vi "ReadWrite.vi"(6 "Values":dbl[](array[numeric]), 7 "tdms file in":refnum<k34>, 8 "error in (no error)":errorcluster, 9 "Channel Refs":T1[](array[typedef]) format="%.0x", 10 "Wfm Refs":refnum<class "Single Waveform Read (DBL).lvclass">[](array[class]), 11 "Compiled.Settings":T2={"Name"="", "Async Init Timeout"=0, "File Data"={"Date Captured"="", "Directory"="", "Name"="", "Groups"=[], "Meta Data"=[]}, "Segment Files"=FALSE, "Segment Every"=0.0, "Trigger?"=FALSE, "Segment by"=enum."Size (MB)", "Trigger Ref"=0} {"Trigger Ref" format="%.0x"; "File Data"."Groups"."Channels"."Data Reference in" format="%.0x"}) -> (0 "error out":errorcluster, 1 "Bytes Written":u64, 2 "tdms file out":refnum<k34>, 3 "Compiled.Settings Out":T2={"Name"="", "Async Init Timeout"=0, "File Data"={"Date Captured"="", "Directory"="", "Name"="", "Groups"=[], "Meta Data"=[]}, "Segment Files"=FALSE, "Segment Every"=0.0, "Trigger?"=FALSE, "Segment by"=enum."Size (MB)", "Trigger Ref"=0} {"Trigger Ref" format="%.0x"; "File Data"."Groups"."Channels"."Data Reference in" format="%.0x"})   [LabVIEW 2023, in "Embedded TDMS Logger Engine.lvlib"]
uses:
  Embedded TDMS Logger Engine.lvlib
  Shared/Compiled.Settings.ctl
  Shared/FileData.ctl
  Shared/GroupData.ctl
  Shared/Meta Data Item.ctl
  Shared/ChannelData.ctl
  <vilib>/NI VeriStand/Custom Device API/Data Reference.ctl
  Shared/SegmentOptions.ctl
  <vilib>/NI VeriStand/Custom Device Waveform API/Single Waveform Read (DBL)/Single Waveform Read (DBL).lvclass
  C:/Program Files/National Instruments/LabVIEW 2023/vi.lib/NI VeriStand/Custom Device Waveform API/Waveform Session.lvclass
  <vilib>/NI VeriStand/Custom Device Waveform API/Waveform Session.lvclass/Waveform Session.ctl
  <vilib>/NI VeriStand/Custom Device Waveform API/Single Waveform Read (DBL)/Single Waveform Read (DBL).lvclass/Single Waveform Read (DBL).ctl
  <vilib>/NI VeriStand/Custom Device Waveform API/Internal Comm Classes/WPL Comm/WPL Comm (1D DBL)/WPL Comm (1D DBL).lvclass/WPL Comm (1D DBL).ctl
  <vilib>/NI VeriStand/Custom Device Waveform API/Single Waveform Read (DBL)/NI VeriStand - Read Single Waveform (DBL).vi
  <vilib>/NI VeriStand/Custom Device Waveform API/Internal Comm Classes/WPL Comm/WPL Comm (1D DBL)/Comm_read 1d dbl.vi
  <vilib>/NI VeriStand/Custom Device Waveform API/Check Opened.vi
  <vilib>/NI VeriStand/Custom Device Waveform API/Internal Comm Classes/WPL Comm/Convert Q Error to Shutdown Error.vi
  <vilib>/Utility/error.llb/Error Cluster From Error Code.vi
  <vilib>/NI VeriStand/Custom Device Waveform API/NI_VS Custom Device Waveform API.lvlib
  Shared/Embedded TDMS Logger Shared.lvlib
  <vilib>/NI VeriStand/Custom Device API/Custom Device API.lvlib
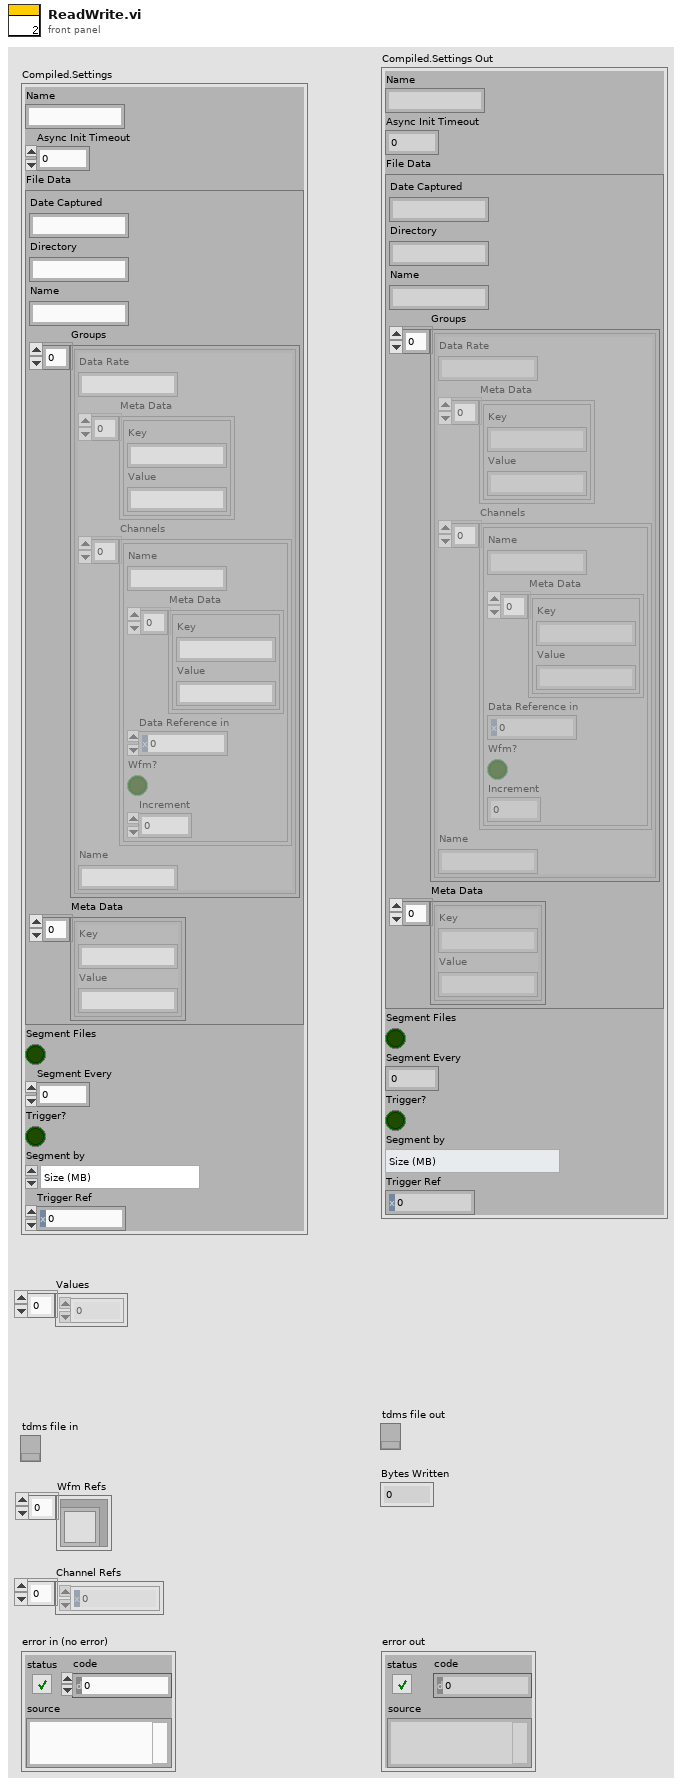
[diagram p1: front panel]
types:
  T1 = typedef "Custom Device API.lvlib/Data Reference.ctl" = i32
  T2 = typedef "Embedded TDMS Logger Shared.lvlib/Compiled.Settings.ctl" = cluster{"Name":string, "Async Init Timeout":u16, "File Data":T3, "Segment Files":bool, "Segment Every":dbl, "Trigger?":bool, "Segment by":T7, "Trigger Ref":T1}
  T3 = typedef "Embedded TDMS Logger Shared.lvlib/FileData.ctl" = cluster{"Date Captured":string, "Directory":string, "Name":string, "Groups":T4[], "Meta Data":T5[]}
  T4 = typedef "Embedded TDMS Logger Shared.lvlib/GroupData.ctl" = cluster{"Data Rate":string, "Meta Data":T5[], "Channels":T6[], "Name":string}
  T5 = typedef "Embedded TDMS Logger Shared.lvlib/Meta Data Item.ctl" = cluster{"Key":string, "Value":string}
  T6 = typedef "Embedded TDMS Logger Shared.lvlib/ChannelData.ctl" = cluster{"Name":string, "Meta Data":T5[], "Data Reference":T1, "Wfm?":bool, "Increment":dbl}
  T7 = typedef "SegmentOptions.ctl" = enum16{"Time (s)", "Size (MB)"}
  T8 = typedef "NI_VS Custom Device Waveform API.lvlib/Waveform properties.ctl" = cluster{"Data reference":T9, "t0 at start":timestamp, "dt":dbl, "offset from start (samples)":u64}
  T9 = typedef "Custom Device API.lvlib/Waveform Data Reference.ctl" = i32
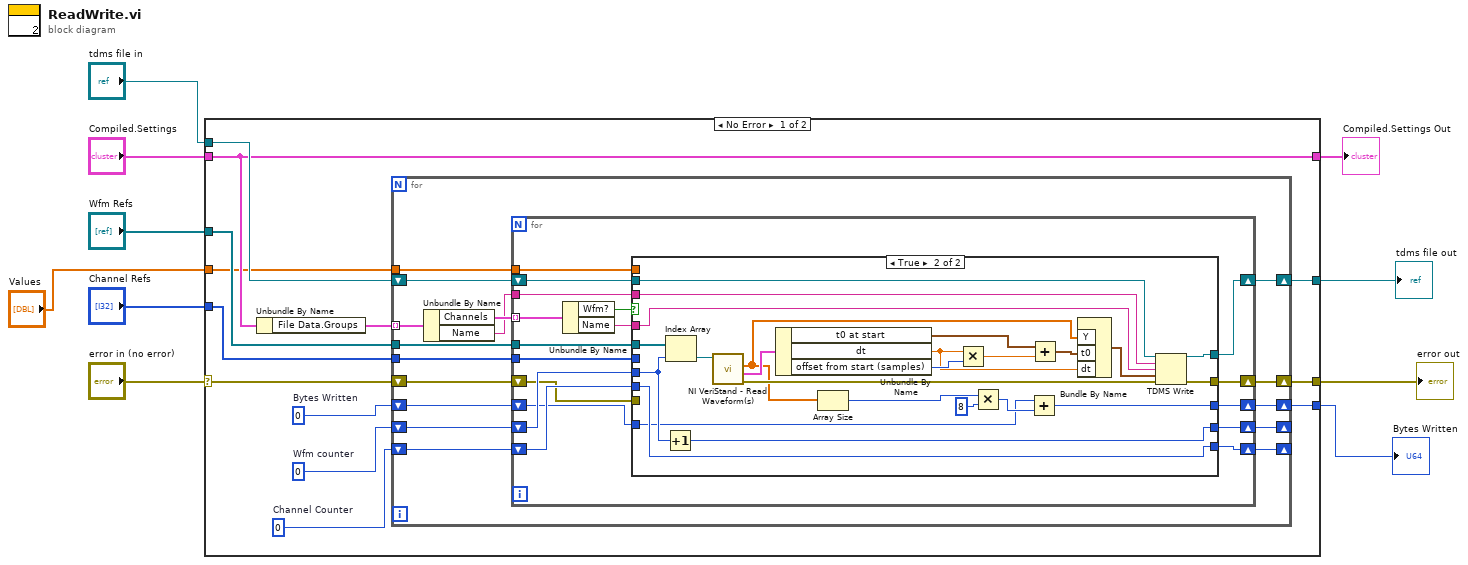
[diagram p0: block diagram]
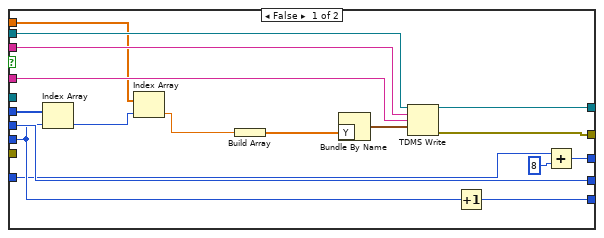
[diagram p2: hidden frame]
diagram:
  n1 = case shown="No Error" "error in (no error)" {
    selector: "error in (no error)" -> [w16 w99]
    tunnel: "Compiled.Settings" -> [w14 w98]
    tunnel: "tdms file in" -> [w22 w100]
    tunnel: [w21 w100] -> w7
    tunnel: "Wfm Refs" -> [w20 _]
    tunnel: "Channel Refs" -> [w17 _]
    tunnel: [w15 w99] -> w4
    tunnel: [w14 w98] -> w3
    tunnel: [w12 _] -> w2
    tunnel: "Values" -> [w11 _]
    frame No Error {
      w13 = u64 0  # Bytes Written
      w19 = 0  # Wfm counter
      w18 = 0  # Channel Counter
      n2 = Unbundle By Name(w14) -> ("File Data.Groups"=w23:T4[])
      n3 = for {
        tunnel: w23 -> [w39] mode=indexing
        shift-right: [w29] -> w21
        shift-left: w22 -> [w36]
        tunnel: w20 -> [w35]
        shift-right: [w32] -> _
        shift-left: w19 -> [w34]
        shift-right: [w31] -> _
        shift-left: w18 -> [w33]
        tunnel: w17 -> [w30]
        shift-right: [w28] -> w15
        shift-left: w16 -> [w27]
        shift-right: [w25] -> w12
        shift-left: w13 -> [w26]
        tunnel: w11 -> [w24]
        n4 = Unbundle By Name(w39) -> ("Channels"=w38:T6[], "Name"=w37:string)
        n5 = for {
          tunnel: w38 -> [w56] mode=indexing
          tunnel: w37 -> [w47]
          shift-right: [w45] -> w29
          shift-left: w36 -> [w54]
          tunnel: w35 -> [w53]
          shift-right: [w50] -> w32
          shift-left: w34 -> [w52]
          shift-right: [w49] -> w31
          shift-left: w33 -> [w51]
          tunnel: w30 -> [w48]
          shift-right: [w44] -> w28
          shift-left: w27 -> [w43]
          shift-right: [w41] -> w25
          shift-left: w26 -> [w42]
          tunnel: w24 -> [w40]
          n6 = Unbundle By Name(w56) -> ("Wfm?"=w55:bool, "Name"=w46:string)
          n7 = case shown="True" w55 {
            tunnel: w54 -> [w70 w97]
            tunnel: w53 -> [_ w95]
            tunnel: w52 -> [w73 w94]
            tunnel: w51 -> [w64 w92]
            tunnel: [w73 w93] -> w50
            tunnel: [w72 w92] -> w49
            tunnel: w48 -> [w71 _]
            tunnel: w47 -> [w69 w82]
            tunnel: w46 -> [w65 w81]
            tunnel: [w68 w90] -> w45
            tunnel: [w67 w91] -> w44
            tunnel: w43 -> [_ _]
            tunnel: w42 -> [w62 w78]
            tunnel: [w61 w77] -> w41
            tunnel: w40 -> [w58 _]
            frame False {
              n8 = Index Array(array=w71, index=w64) -> (element=w60:T1)
              n9 = Index Array(array=w58, index=w60) -> (element=w59:dbl)
              n10 = Build Array(w59) -> (w57:dbl[])
              n11 = Bundle By Name("Y"=w57) -> (w66:waveform(dbl))  [unwired: 1 in]
              n12 = TDMS Write(0:w70, 5:w69, 7:w65, 9:w66) -> (4:w68:refnum<k34>, 15:w67:errorcluster)  [unwired: 2 in, 2 out]
              n13 = Increment(x=w64) -> (x+1=w72:i32)
              n14 = Add(x=w62, y=u64 8) -> (x+y=w61:u64)
            }
            frame True {
              n15 = Increment(x=w94) -> (x+1=w93:i32)
              n16 = Index Array(array=w95, index=w94) -> (element=w96:refnum<class "Single Waveform Read (DBL).lvclass">)
              n17 = call-poly <vilib>:"NI VeriStand - Read Waveform(s).vi"("Single Waveform Read Session (DBL) in"=w96) -> ("error out"=w89:errorcluster, "Properties"=w88:T8, "Data"=w75:dbl[])  [unwired: 6 in, 2 out]
              n18 = Unbundle By Name(w88) -> ("t0 at start"=w76:timestamp, "dt"=w85:dbl, "offset from start (samples)"=w87:u64)
              n19 = Array Size(array=w75) -> (size(s)=w74:i32)
              n20 = Multiply(x=w85, y=w87) -> (x*y=w86:dbl)
              n21 = Multiply(x=w74, y=u64 8) -> (x*y=w79:u64)
              n22 = Add(x=w78, y=w79) -> (x+y=w77:u64)
              n23 = Add(x=w76, y=w86) -> (x+y=w84:timestamp)
              n24 = Bundle By Name("Y"=w75, "t0"=w84, "dt"=w85) -> (w83:waveform(dbl))  [unwired: 1 in]
              n25 = TDMS Write(0:w97, 5:w82, 7:w81, 9:w83, 11:w89) -> (4:w90:refnum<k34>, 15:w91:errorcluster)  [unwired: 1 in, 2 out]
            }
          }
        }
      }
    }
    frame Error {
    }
  }
  "error out" <- w4
  "Compiled.Settings Out" <- w3
  "tdms file out" <- w7
  "Bytes Written" <- w2
